vi "POST_error_input.vi"(8 "API Key":string="0", 11 "JSON_input":string="0") -> (0 "headers":string="0\r\nContent-Length: 58\r\nConnection: close\r\n\r\n", 1 "body":string="0", 3 "JSON string":string="0")   [LabVIEW 2024]
uses:
  <vilib>/httpClient/LabVIEWHTTPClient.lvlib
  <vilib>/httpClient/POSTBuffer.vi
panel:
  out "error out put":errorcluster
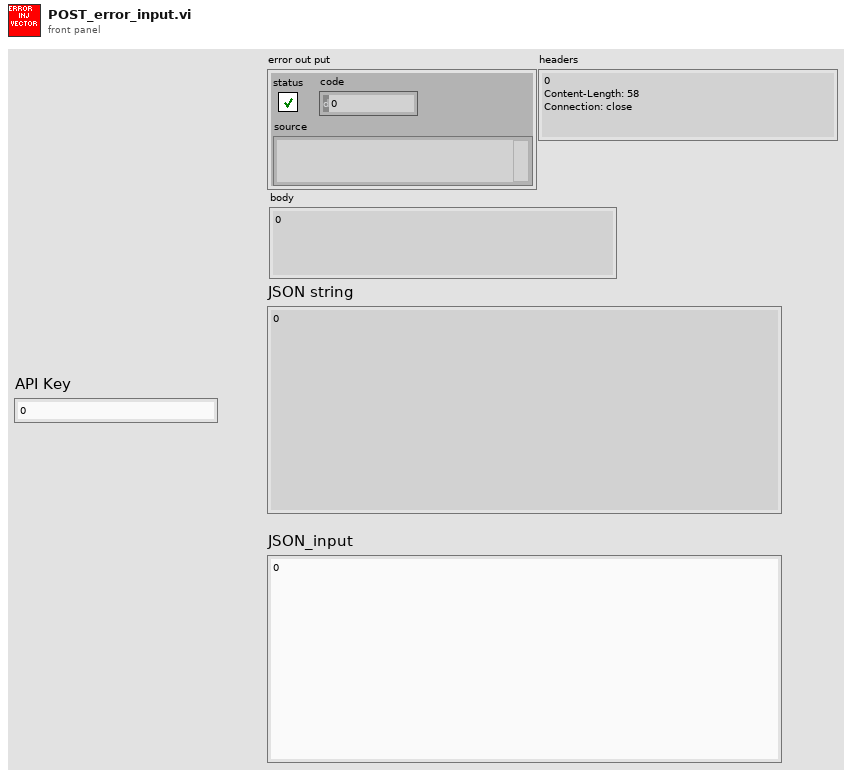
[diagram p1: front panel]
types:
  T1 = typedef "LabVIEWHTTPClient.lvlib/ClientHandle.ctl" = refnum<k1>
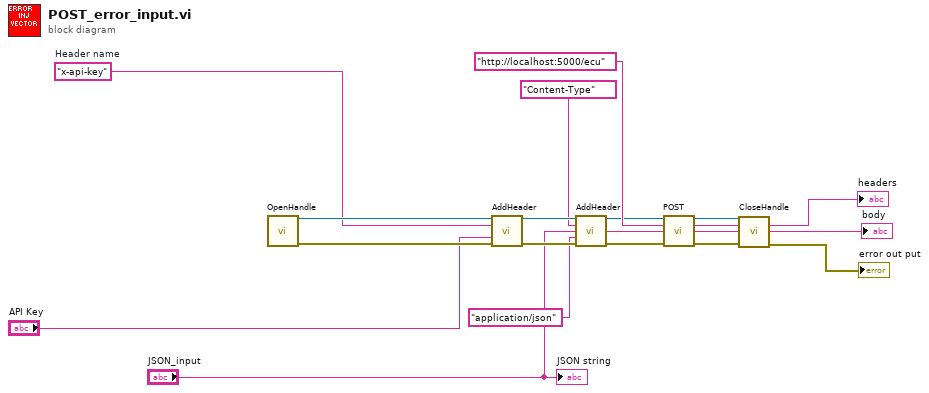
[diagram p0: block diagram]
diagram:
  w10 = "x-api-key"  # Header name
  n1 = call <vilib>:"OpenHandle.vi"() -> ("client handle out"=w11:T1, "error out"=w12:errorcluster)  [unwired: 14 in]
  n2 = call <vilib>:"AddHeader.vi"("client handle"=w11, "header"=w10, "value"="API Key", "error in (no error)"=w12) -> ("client handle out"=w7:T1, "error out"=w4:errorcluster)  [unwired: 10 in]
  n3 = call <vilib>:"AddHeader.vi"("client handle"=w7, "header"="Content-Type", "value"="application/json", "error in (no error)"=w4) -> ("client handle out"=w6:T1, "error out"=w5:errorcluster)  [unwired: 10 in]
  n4 = call-poly <vilib>:"POST.vi"("client handle"=w6, "url"="http://localhost:5000/ecu", "buffer"="JSON_input", "error in (no error)"=w5) -> ("client handle out"=w14:T1, "headers"=→"headers":string, "body"=→"body":string, "error out"=w13:errorcluster)  [unwired: 8 in]
  n5 = call <vilib>:"CloseHandle.vi"("client handle"=w14, "error in (no error)"=w13) -> ("error out"=→"error out put":errorcluster)  [unwired: 13 in]
  "JSON string" <- "JSON_input"
